vi "RoomNo.vi"(8 "error in (no error)":errorcluster, 10 "RoomNumber":i32, 11 "Maze in":refnum<class "Maze.lvclass">) -> (0 "error out":errorcluster, 2 "Room":refnum<class "Room.lvclass">, 3 "Maze out":refnum<class "Maze.lvclass">)   [LabVIEW 2020, in "Maze.lvclass"]
uses:
  Maze.lvclass
  ConcreteMazeSite/Room/Room.lvclass
  Maze.lvclass/Maze.ctl
  ConcreteMazeSite/Room/Room.lvclass/Room.ctl
  ConcreteMazeSite/Room/Property/roomNumber/Read roomNumber.vi
  Private/Property/mRoomVec/Read mRoomVec.vi
  MazeSite/MazeSite.lvclass
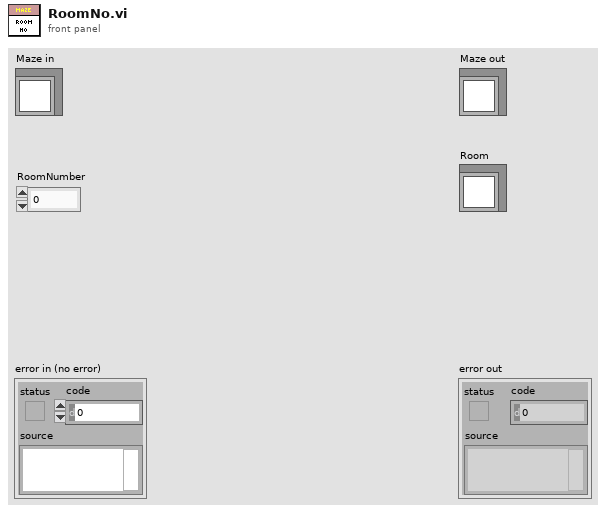
[diagram p1: front panel]
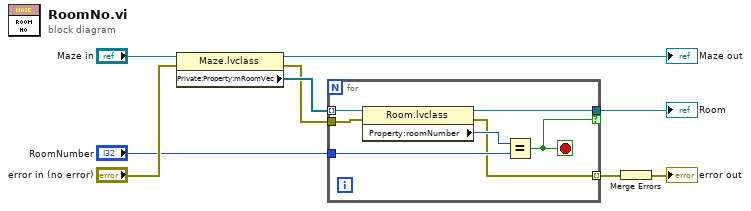
[diagram p0: block diagram]
diagram:
  n1 = property class="Maze.lvclass"(reference="Maze in", error in="error in (no error)") -> (reference out=→"Maze out":refnum<class "Maze.lvclass">, error out=w4:errorcluster, "Private:Property:mRoomVec"=w5:refnum<class "Room.lvclass">[])
  n2 = for {
    tunnel: w5 -> [w16] mode=indexing
    tunnel: "RoomNumber" -> [w14]
    tunnel: [w13] -> w1 if=w12
    tunnel: w4 -> [w11]
    tunnel: [w10] -> w3 mode=indexing
    stop <- w12 stop-if-true
    n3 = property class="Room.lvclass"(reference=w16, error in=w11) -> (reference out=w13:refnum<class "Room.lvclass">, error out=w10:errorcluster, "Property:roomNumber"=w15:i32)
    n4 = Equal?(x=w15, y=w14) -> (x = y?=w12:bool)
  }
  "Room" <- w1
  n5 = Merge Errors(w3) -> (→"error out":errorcluster)
